vi "LJ-T7DAQ.vi"() -> (0 "Error Out":errorcluster)   [LabVIEW 2020]
uses:
  Globals/Meas_global.vi
  ADAM Serial/Instrument drivers/LabJack/T7/Stream/T7 Stream Globals KAG.vi
  ADAM Serial/Instrument drivers/LabJack/T7/Stream/T7 Stream Config KAG.ctl
  Sub_vis/Upload Data.ctl
panel:
  in  "Tab Control":enum32{"Page 1", "Page 2"}(tab)
  out "input terminal configuration":i32(ring)=10106 items=["default"=-1, "RSE"=10083, "NRSE"=10078, "Differential"=10106, "Pseudodifferential"=12529]
  out "AuditTrail":string[](array[string])
  out "Waveform Graph":dbl[][](graph)
  in  "milliseconds holdup":u32
  out "Requested # Blks":i32
  out "Current Block No":i32
  out "Strm Config Out":T1={"Scan Rate (Hz)"=1000.0, "Samples Per Packet"=512, "Resolution Index"=0, "Buffer Size (bytes)"=32768, "NumScans"=1500, "Read Timeout (ms)"=5000, "Scan Table"=[{"Channel"=0, "BipGain"=0, "Input Config"="Single-Ended"}, {"Channel"=1, "BipGain"=0, "Input Config"="Single-Ended"}, {"Channel"=2, "BipGain"=0, "Input Config"="Single-Ended"}, {"Channel"=3, "BipGain"=0, "Input Config"="Single-Ended"}]} {"Samples Per Packet" max=512 step=1; "Buffer Size (bytes)" max=32768 step=1; "Resolution Index" max=8 step=1; "Scan Rate (Hz)" max=100000; "Scan Table"."BipGain" items=["x1", "x10", "x100", "x1000"]; "Scan Table"."Channel" step=1}
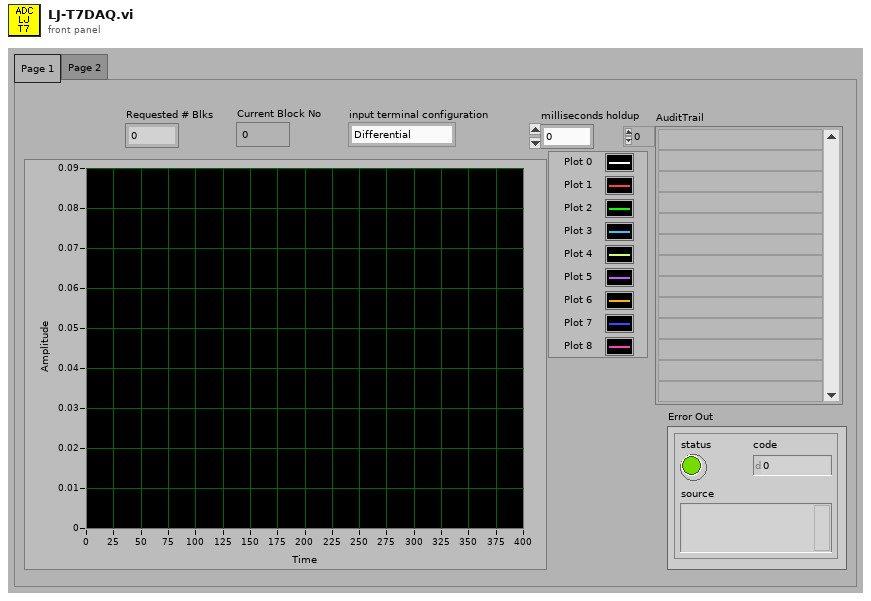
[diagram p1: front panel]
types:
  T1 = typedef "T7 Stream Config KAG.ctl" = cluster{"Scan Rate (Hz)":sgl, "Samples Per Packet":u32, "Resolution Index":u32, "Buffer Size (bytes)":u32, "NumScans":u32, "Read Timeout (ms)":u32, "Scan Table":cluster{"Channel":u32, "BipGain":u32, "Input Config":string}[]}
  T2 = typedef "Analysis_info_cluster.ctl" = cluster{"Colour":u32, "Inst type":T3, "Inst name":string, "Symbol":string, "Code name":string, "Extra Info":string, "Inst Array":T4, "Extra Titles":string[], "Extra Values":string[], "U":dbl, "u^2":dbl, "u^3":dbl, "u^4":dbl, "Skew_u":dbl, "Kurt_u":dbl, "Sd Error in Mean":dbl, "% u'/U":dbl, "X":dbl, "Y":dbl, "Z":dbl, "Timescale integral Estimate":dbl, "Sd Error in Variance":dbl, "Calib File":path, "Calib Constants":dbl[], "Output Position":bool, "Stats":enum16{"None", "Basic", "Full"}, "Av Sampling Rate":dbl, "Av No of Samples":dbl, "Total Meas Time (s)":dbl, "ADAM Ch Name":string, "Max value":dbl, "Min value":dbl, "Req Sample Rate Hz":dbl, "Sync Delay Time (s)":dbl, "Ch No":i16, "Device":string, "Use Latest Calib":bool, "Port":string, "Metadata Ch Names":string[], "Metadata Ch Values":string[], "Label":string}
  T3 = typedef "Inst_type.ctl" = enum16{"Raw voltage", "Raw with zero offsetting", "Propeller anemometer", "Pressure Transducer", "Pitot-static tube", "Hot wire", "Cross wire 1", "Cross wire 2", "Generic Linear", "Generic Polynomial", "Generic BackPoly", "Fast FID", "Thermocouple", "Cold wire", "Pulsed Wire", "LDA Vel", "LDA Tran time", "LDA Arr time", "Microphone"}
  T4 = typedef "Instrument_Array.ctl" = enum16{"PWA", "LDA", "Analogue"}
  T5 = typedef "Device ID port info.ctl" = cluster{"Ch No":i16[], "Req Sampling Rate":dbl[], "Port":string, "Index":i32[]}
  T6 = typedef "Upload Data.ctl" = enum16{"Voltage Array", "Time Trace Cluster"}
  T7 = typedef "Setup.ctl" = enum16{"Run Program", "Show Setup", "Save Current Setup", "Setup Front Panel"}
  T8 = cluster{"PSlope":dbl, "NSlope":dbl, "AvgSlope":dbl, "Center":dbl, "Offset":dbl}[]
  T9 = cluster{"Channel":u32, "BipGain":u32, "Input Config":string}[]
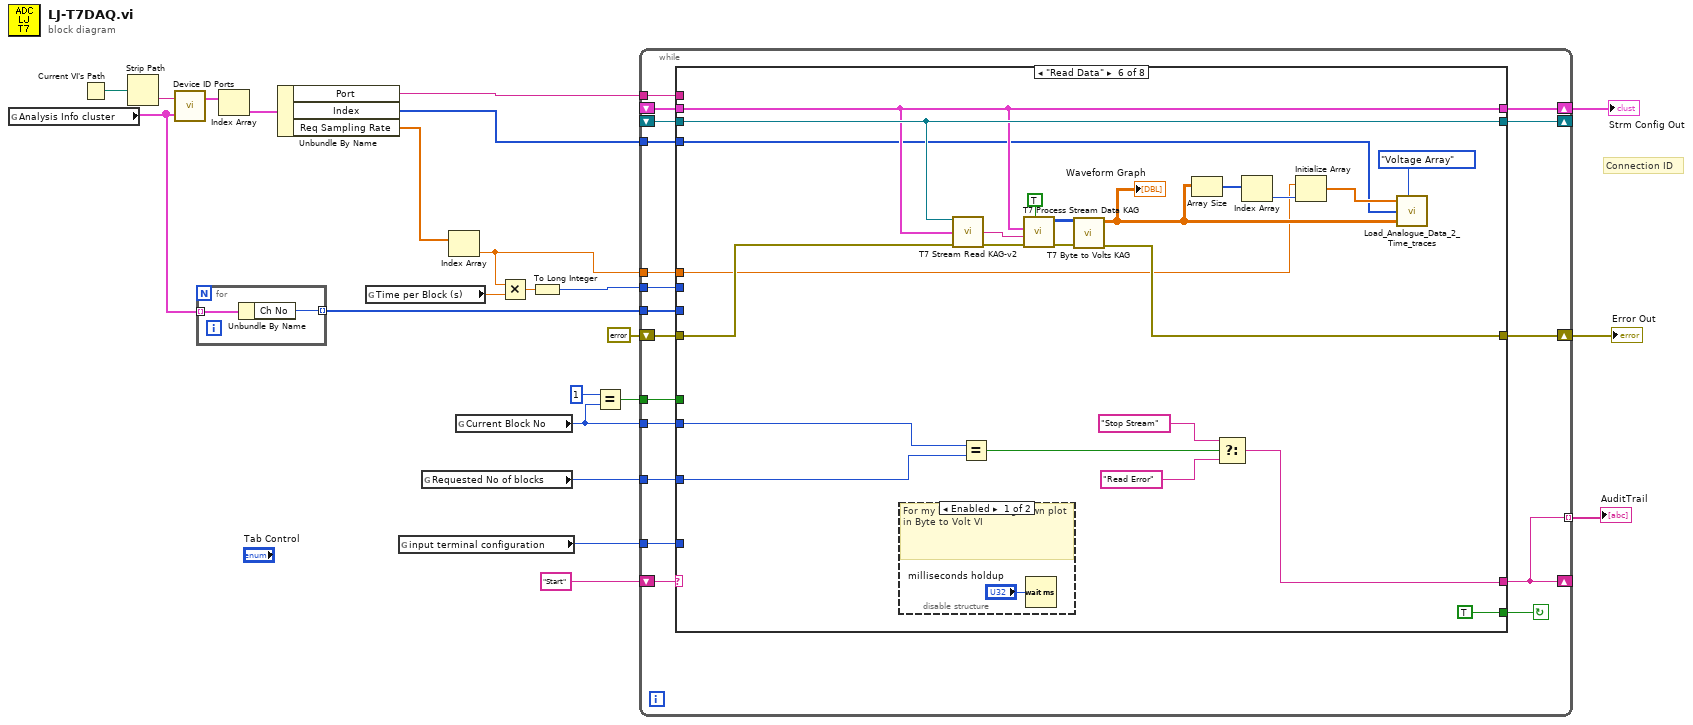
[diagram p0: block diagram]
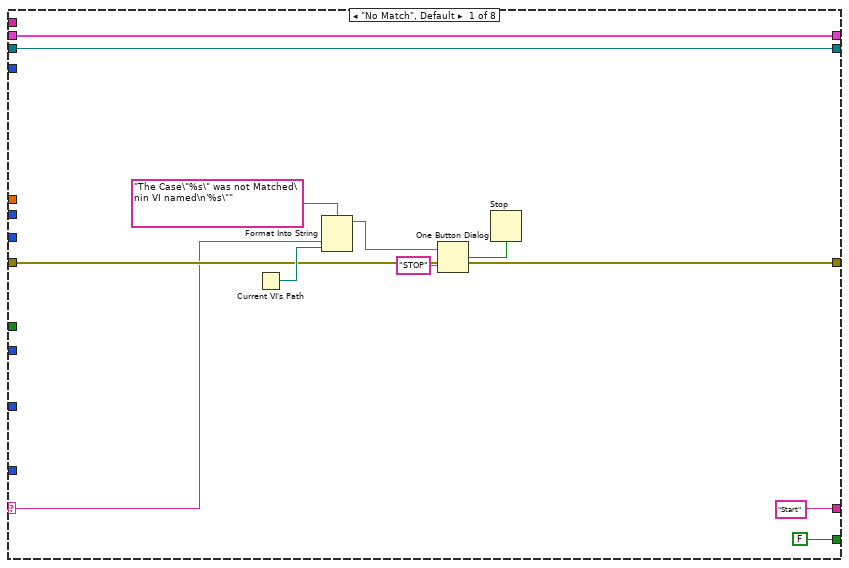
[diagram p2: hidden frame]
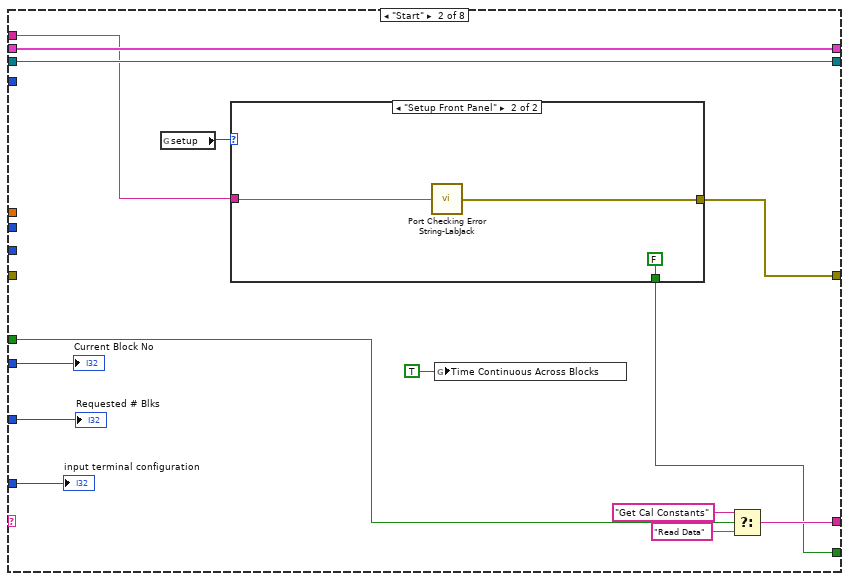
[diagram p3: hidden frame]
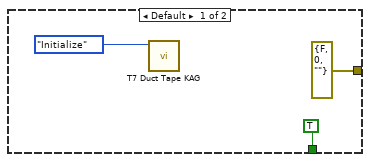
[diagram p4: hidden frame]
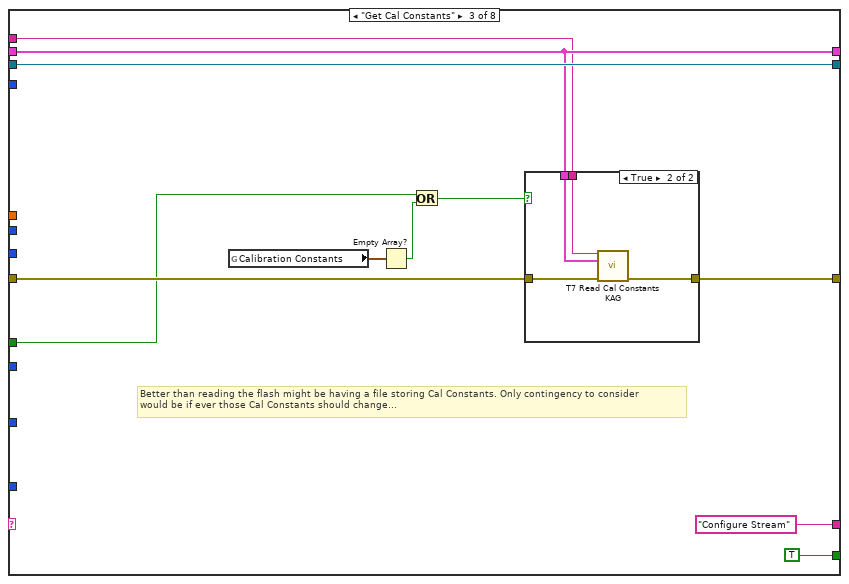
[diagram p5: hidden frame]
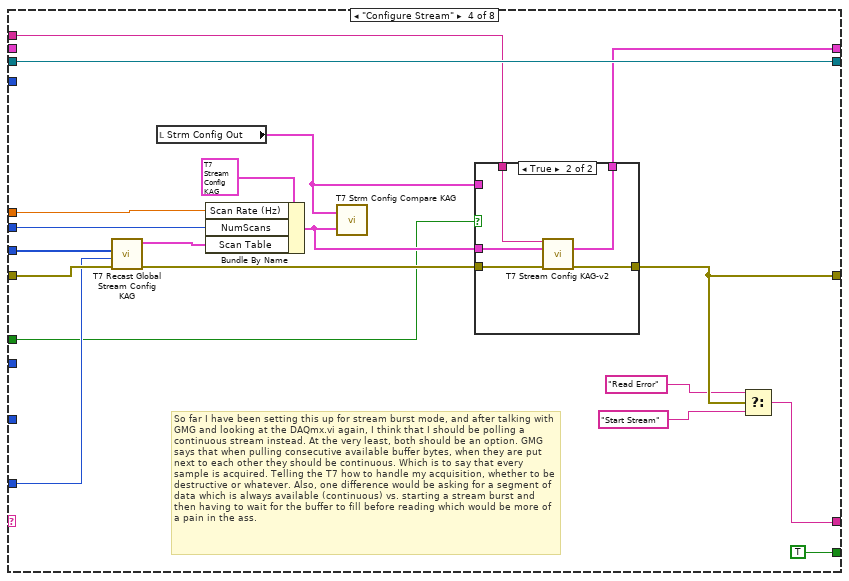
[diagram p7: hidden frame]
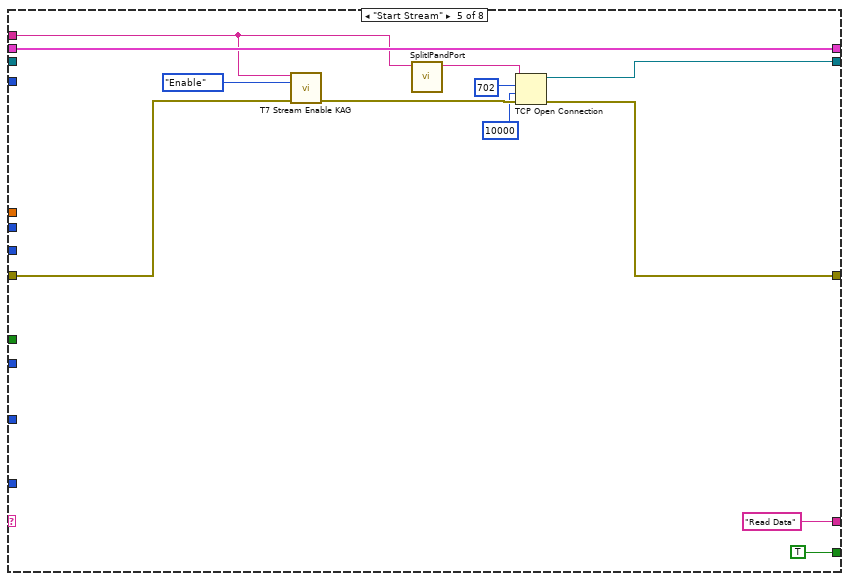
[diagram p9: hidden frame]
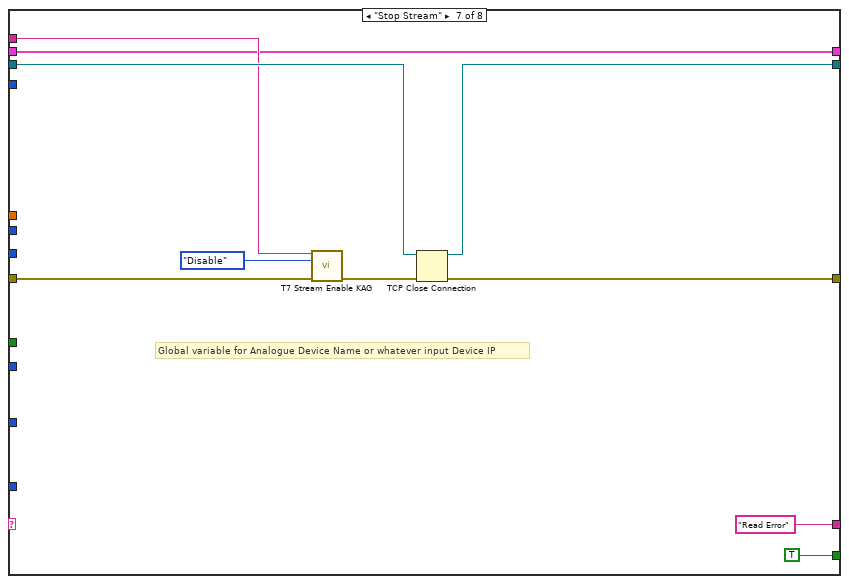
[diagram p11: hidden frame]
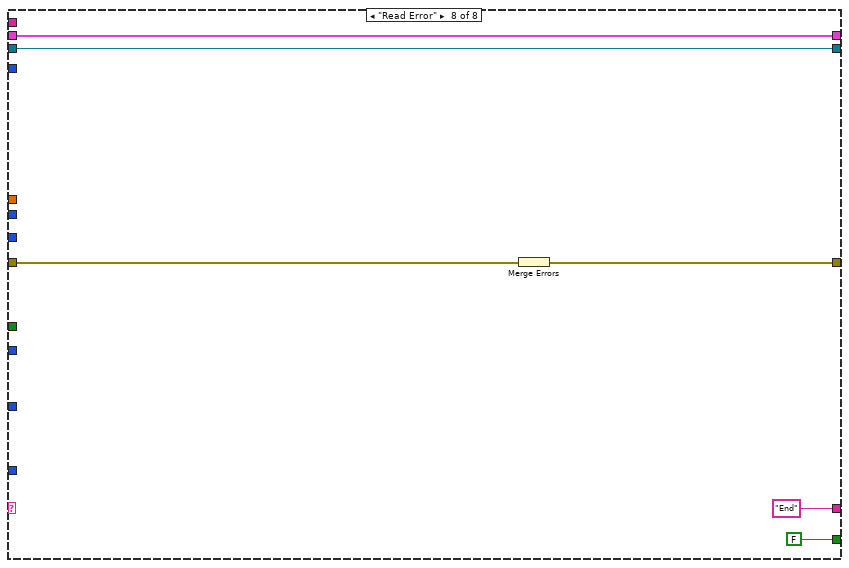
[diagram p12: hidden frame]
diagram:
  # "Connection ID"
  n1 = global read "Meas_global.vi" "Analysis Info cluster"() -> (w7:T2[])
  n2 = Current VI's Path() -> (path=w12:path)
  n3 = Strip Path(path=w12) -> (name=w13:string)  [unwired: 1 out]
  n4 = call "Device ID Ports.vi"("Analysis Info cluster"=w7, "Device ID"=w13) -> ("Device port info"=w14:T5[])  [unwired: 1 out]
  n5 = for {
    tunnel: w7 -> [w25] mode=indexing
    tunnel: [w24] -> w6 mode=indexing
    n6 = Unbundle By Name(w25) -> ("Ch No"=w24:i16)
  }
  n7 = Index Array(array=w14) -> (element=w15:T5)  [unwired: 1 in]
  n8 = Unbundle By Name(w15) -> ("Port"=w4:string, "Index"=w5:i32[], "Req Sampling Rate"=w16:dbl[])
  n9 = global read "Meas_global.vi" "Time per Block (s)"() -> (w10:dbl)
  n10 = global read "Meas_global.vi" "input terminal configuration"() -> (w21:i32)
  n11 = global read "Meas_global.vi" "Requested No of blocks"() -> (w19:i32)
  n12 = Index Array(array=w16) -> (element=w9:dbl)  [unwired: 1 in]
  n13 = global read "Meas_global.vi" "Current Block No"() -> (w3:i32)
  n14 = Multiply(x=w9, y=w10) -> (x*y=w11:dbl)
  n15 = To Long Integer(number=w11) -> (32bit integer=w8:i32)
  n16 = Equal?(x=1, y=w3) -> (x = y?=w1:bool)
  n17 = while {
    shift-left: "Start" -> [w42]
    shift-right: [w36] -> _
    shift-right: [w37] -> w17
    shift-left: errorcluster {"status"=FALSE, "code"=0, "source"=""} ("error IO") -> [w41]
    tunnel: w9 -> [w40]
    tunnel: w8 -> [w39]
    tunnel: [w36] -> w22 mode=indexing
    shift-right: [w35] -> _
    shift-left: _ -> [w34]
    shift-right: [w33] -> w18
    shift-left: _ -> [w32]
    tunnel: w21 -> [w31]
    tunnel: w19 -> [w30]
    tunnel: w3 -> [w38]
    tunnel: w6 -> [w29]
    tunnel: w5 -> [w28]
    tunnel: w4 -> [w27]
    tunnel: w1 -> [w26]
    stop <- w43 continue-if-true
    n18 = case shown="\"Read Data\"" w42 {
      selector: w42 -> [w46 _ _ _ _ _ _ _]
      tunnel: [FALSE w57 TRUE TRUE TRUE TRUE TRUE FALSE] -> w43
      tunnel: ["Start" w61 "Configure Stream" ("f") w100 "Read Data" w145 "Read Error" "End" ("f")] -> w36
      tunnel: [w47 w55 w84 w103 w122 w147 w156 w167] -> w37
      tunnel: w41 -> [w47 _ w85 w108 w126 w146 w160 w168]
      tunnel: w40 -> [_ _ _ w98 _ w131 _ _]
      tunnel: w39 -> [_ _ _ w97 _ _ _ _]
      tunnel: w38 -> [_ w64 _ _ _ w138 _ _]
      tunnel: [w45 w68 w81 w106 w119 w143 w158 w164] -> w35
      tunnel: w34 -> [w45 w68 w81 w106 _ w143 w159 w164]
      tunnel: w27 -> [_ w56 w76 w105 w118 _ w155 _]
      tunnel: [w44 w67 w80 w99 w125 w142 w154 w163] -> w33
      tunnel: w32 -> [w44 w67 w80 _ w125 w142 w154 w163]
      tunnel: w31 -> [_ w66 _ w104 _ _ _ _]
      tunnel: w30 -> [_ w65 _ _ _ w137 _ _]
      tunnel: w29 -> [_ _ _ w92 _ _ _ _]
      tunnel: w28 -> [_ _ _ _ _ w130 _ _]
      tunnel: w26 -> [_ w59 w75 w91 _ _ _ _]
      frame "No Match", Default {
        n19 = Current VI's Path() -> (path=w49:path)
        n20 = Format Into String(format string="The Case\"%s\" was not Matched\nin VI named\n'%s\"" ("Format String"), w46, w49) -> (resulting string=w52:string)  [unwired: 2 in, 1 out]
        n21 = One Button Dialog(message=w52, button name ("OK")="STOP") -> (true=w50:bool)
        n22 = Stop(stop? (T)=w50) -> ()
      }
      frame "Start" {
        n23 = global read "Meas_global.vi" "setup"() -> (w58:T7)
        n24 = case shown="\"Setup Front Panel\"" w58 {
          tunnel: w56 -> [_ w74]
          tunnel: [errorcluster {"status"=FALSE, "code"=0, "source"=""} ("error out") w73] -> w55
          tunnel: [TRUE FALSE] -> w57
          frame Default {
            n25 = call "T7 Duct Tape KAG.vi"("Action"=enum16{"Initialize", "Read", "Update"}."Initialize") -> ()  [unwired: 8 in, 1 out]
          }
          frame "Setup Front Panel" {
            n26 = call "Port Checking Error String-LabJack.vi"("Port"=w74) -> ("error out"=w73:errorcluster)  [unwired: 3 in]
          }
        }
        n27 = global write "Meas_global.vi" "Time Continuous Across Blocks"(TRUE ("Time Continuous Across Blocks")) -> ()
        n28 = Select(t="Get Cal Constants", s=w59, f="Read Data") -> (s? t:f=w61:string)
        "input terminal configuration" <- w66
        "Requested # Blks" <- w65
        "Current Block No" <- w64
      }
      frame "Get Cal Constants" {
        # "Better than reading the flash might be having a file storing Cal Constants. Only contingency to consider\nwould be if ever those Cal Constants should change..."
        n29 = global read "T7 Stream Globals KAG.vi" "Calibration Constants"() -> (w79:T8)
        n30 = Empty Array?(array=w79) -> (empty?=w78:bool)
        n31 = Or(x=w75, y=w78) -> (x .or. y?=w77:bool)
        n32 = case shown="True" w77 {
          tunnel: w85 -> [w86 w90]
          tunnel: [w86 w89] -> w84
          tunnel: w76 -> [_ w88]
          tunnel: w80 -> [_ w87]
          frame False {
          }
          frame True {
            n33 = call "T7 Read Cal Constants KAG.vi"("IP:Port"=w88, "Stream Configuration"=w87, "error in"=w90) -> ("error out"=w89:errorcluster)  [unwired: 11 in, 1 out]
          }
        }
      }
      frame "Configure Stream" {
        # "So far I have been setting this up for stream burst mode, and after talking with GMG and looking at the DAQmx.vi again, I think that I should be polling a continuous stream instead. At the very least, both should be an option. GMG says that when pulling consecutive available buffer bytes, when they are put next to each other they should be continuous. Which is to say that every sample is acquired. Telling the T7 how to handle my acquisition, whether to be destructive or whatever. Also, one difference would be asking for a segment of data which is always available (continuous) vs. starting a stream burst and then having to wait for the buffer to fill before reading which would be more of a pain in the ass."
        n34 = call "T7 Recast Global Stream Config KAG.vi"("error in"=w108, "input terminal configuration"=w104, "Channels"=w92) -> ("error out"=w107:errorcluster, "Scan Table"=w96:T9)  [unwired: 3 in]
        n35 = local read "Strm Config Out"() -> (w93:T1)
        n36 = Bundle By Name(cluster=T1 {"Scan Rate (Hz)"=1000.0, "Samples Per Packet"=512, "Resolution Index"=0, "Buffer Size (bytes)"=32768, "NumScans"=1500, "Read Timeout (ms)"=5000, "Scan Table"=[{"Channel"=0, "BipGain"=0, "Input Config"="Single-Ended"}, {"Channel"=1, "BipGain"=0, "Input Config"="Single-Ended"}, {"Channel"=2, "BipGain"=0, "Input Config"="Single-Ended"}, {"Channel"=3, "BipGain"=0, "Input Config"="Single-Ended"}]} ("Stream Configuration"), "Scan Rate (Hz)"=w98, "NumScans"=w97, "Scan Table"=w96) -> (w94:T1)
        n37 = call "T7 Strm Config Compare KAG.vi"("Strm Config 1"=w94, "Strm Config 2"=w93) -> ()  [unwired: 1 out]
        n38 = case shown="True" w91 {
          tunnel: w107 -> [w111 w116]
          tunnel: w105 -> [_ w112]
          tunnel: [w111 w115] -> w103
          tunnel: [w110 w114] -> w99
          tunnel: w94 -> [_ w113]
          tunnel: w93 -> [w110 _]
          frame False {
          }
          frame True {
            n39 = call "T7 Stream Config KAG-v2.vi"("IP:Port"=w112, "Stream Configuration"=w113, "error in"=w116) -> ("Strm Config Out"=w114:T1, "error out"=w115:errorcluster)  [unwired: 11 in]
          }
        }
        n40 = Select(t="Read Error", s=w103, f="Start Stream") -> (s? t:f=w100:string)
      }
      frame "Start Stream" {
        n41 = call "T7 Stream Enable KAG.vi"("IP:Port"=w118, "Enable"=enum32{"Disable", "Enable"}."Enable", "error in"=w126) -> ("error out"=w123:errorcluster)  [unwired: 12 in]
        n42 = call "SplitIPandPort.vi"("IP:Port"=w118) -> ("IP"=w117:string)  [unwired: 9 in, 1 out]
        n43 = TCP Open Connection(address=w117, remote port or service name=702 ("Port"), timeout ms (60000)=10000, error in (no error)=w123) -> (connection ID=w119:refnum<k5>, error out=w122:errorcluster)  [unwired: 1 out]
      }
      frame "Read Data" {
        n44 = disable-structure shown="Enabled" {
          frame Enabled {
            # "For my benefit...slowing down plot in Byte to Volt VI"
            n45 = Wait (ms)(milliseconds to wait="milliseconds holdup") -> ()  [unwired: 1 out]
          }
          frame Disabled {
          }
        }
        n46 = call "T7 Stream Read KAG-v2.vi"("Connection ID In"=w143, "Stream Configuration"=w142, "error in"=w146) -> ("TCP Data"=w144:string, "error out"=w150:errorcluster)  [unwired: 10 in, 1 out]
        n47 = Equal?(x=w138, y=w137) -> (x = y?=w136:bool)
        n48 = call "T7 Process Stream Data KAG.vi"("Backlog"=TRUE, "error in"=w150, "TCP Data In"=w144, "Stream Configuration"=w142) -> ("error out"=w149:errorcluster, "Data"=w148:u16[][])  [unwired: 4 in, 2 out]
        n49 = call "T7 Byte to Volts KAG.vi"("error in"=w149, "Byte Data"=w148) -> ("error out"=w147:errorcluster, "Float Data"=w135:dbl[][])  [unwired: 8 in]
        "Waveform Graph" <- w135
        n50 = Array Size(array=w135) -> (size(s)=w134:i32[])
        n51 = Select(t="Stop Stream" ("f"), s=w136, f="Read Error") -> (s? t:f=w145:string)
        n52 = Index Array(array=w134) -> (element=w133:i32)  [unwired: 1 in]
        n53 = Initialize Array(w131, w133) -> (w132:dbl[])
        n54 = call "Load_Analogue_Data_2_Time_traces.vi"("Sampling Rate (Hz)"=w132, "Mode"=Upload_Data."Voltage Array", "Index"=w130, "Voltage Array"=w135) -> ()  [unwired: 3 in]
      }
      frame "Stop Stream" {
        # "Global variable for Analogue Device Name or whatever input Device IP"
        n55 = call "T7 Stream Enable KAG.vi"("IP:Port"=w155, "Enable"=enum32{"Disable", "Enable"}."Disable", "error in"=w160) -> ("error out"=w157:errorcluster)  [unwired: 12 in]
        n56 = TCP Close Connection(connection ID=w159, error in (no error)=w157) -> (connection ID out=w158:refnum<k5>, error out=w156:errorcluster)  [unwired: 1 in]
      }
      frame "Read Error" {
        n57 = Merge Errors(w168) -> (w167:errorcluster)
      }
    }
  }
  "AuditTrail" <- w22
  "Strm Config Out" <- w18
  "Error Out" <- w17
